vi "Calculate sleeping line.vi"(8 "error in (no error)":errorcluster, 10 "Pixel density":dbl format="%#_13g", 11 "Input point":cluster{"X":sgl, "Y":sgl}) -> (0 "error out":errorcluster, 1 "Sleeping line start point":cluster{"X":sgl, "Y":sgl}, 2 "slanting line start poing":cluster{"X":sgl, "Y":sgl}, 3 "Angle":sgl)   [LabVIEW 2015]
uses:
  <vilib>/vision/NI_Vision_Development_Module.lvlib
panel:
  out "error out 2":errorcluster
  in  "Line":T1
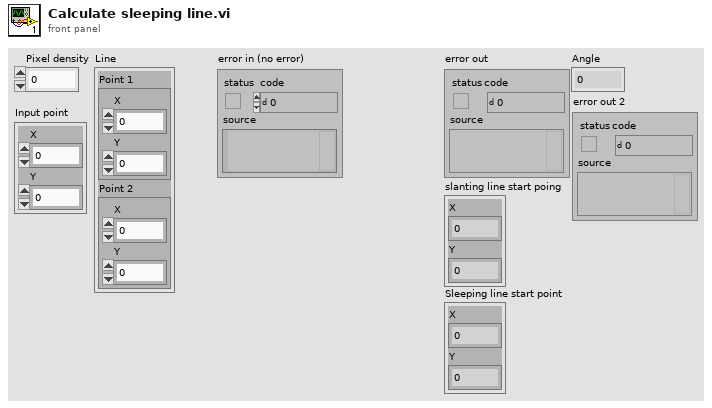
[diagram p1: front panel]
types:
  T1 = cluster{"Point 1":cluster{"X":sgl, "Y":sgl}, "Point 2":cluster{"X":sgl, "Y":sgl}}
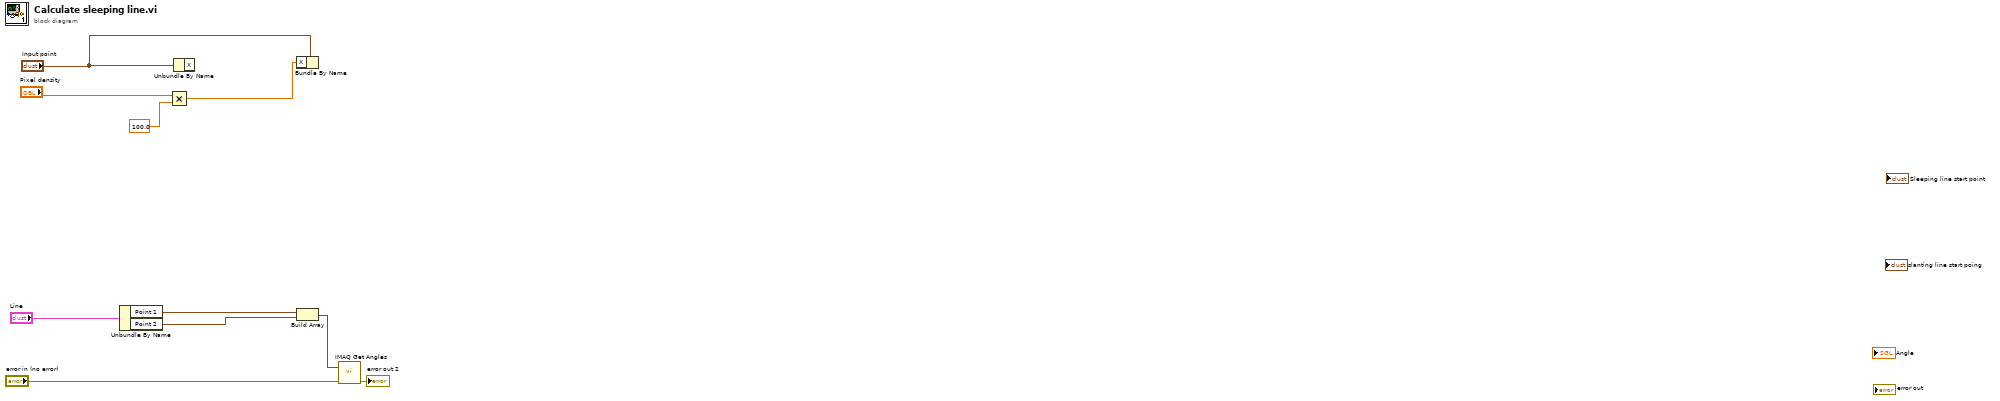
[diagram p0: block diagram]
diagram:
  n1 = Unbundle By Name("Line") -> ("Point 1"=w6:cluster{"X":sgl, "Y":sgl}, "Point 2"=w5:cluster{"X":sgl, "Y":sgl})
  n2 = Multiply(x="Pixel density", y=100.0) -> (x*y=w2:dbl)
  n3 = Unbundle By Name("Input point") -> ()  [unwired: 1 out]
  n4 = Bundle By Name(cluster="Input point", "X"=w2) -> ()  [unwired: 1 out]
  n5 = Build Array(w6, w5) -> (w4:cluster{"X":sgl, "Y":sgl}[])
  n6 = call "IMAQ Get Angles"("error in (no error)"="error in (no error)", "Points"=w4) -> ("error out"=→"error out 2":errorcluster)  [unwired: 3 in, 2 out]
